vi "Configure Load Trigger Template.vi"(8 "error in (no error)":errorcluster, 9 "Arguments ()":string, 10 "Templates (0: ConfigList)":i32(ring) items=["ConfigList", "DurationLoop", "Empty", "GradeBinning", "Keithley2001", "LogicTrigger", "LoopUntilEvent", "SimpleLoop", "SortBinning"], 11 "VISA resource name":refnum<visa-resource-name>) -> (0 "error out":errorcluster, 3 "VISA resource name out":refnum<visa-resource-name>)   [LabVIEW 2020, in "Keithley DMM6500 DAQ6500 Series.lvlib"]
doc: "Load the trigger template with the arguments."
uses:
  <instrlib>/Keithley DMM6500 DAQ6500 Series/Keithley DMM6500 DAQ6500 Series.lvlib
panel:
  # "This VI is obsolete and these functions are \nincorporated in \"Configure Load Trigger Template.vi\""
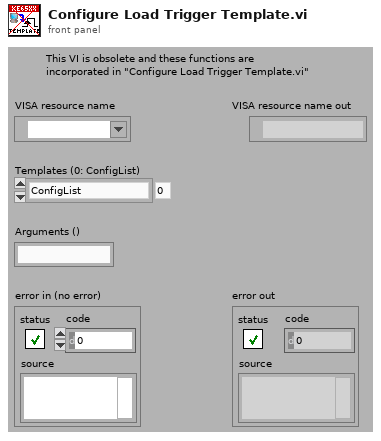
[diagram p1: front panel]
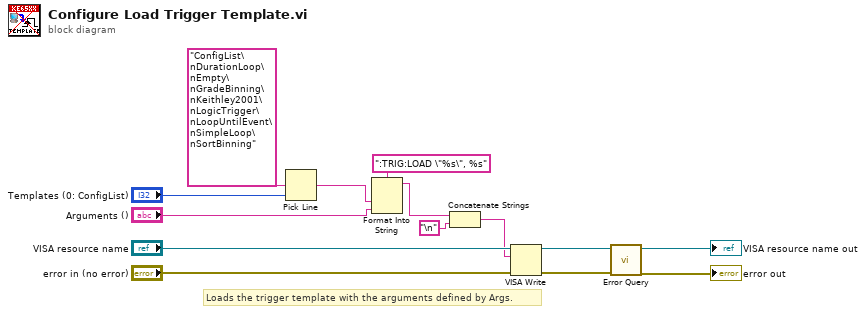
[diagram p0: block diagram]
diagram:
  # "Loads the trigger template with the arguments defined by Args."
  n1 = Pick Line(multi-line string="ConfigList\nDurationLoop\nEmpty\nGradeBinning\nKeithley2001\nLogicTrigger\nLoopUntilEvent\nSimpleLoop\nSortBinning", line index="Templates (0: ConfigList)") -> (output string=w7:string)  [unwired: 1 in]
  n2 = Format Into String(format string=":TRIG:LOAD \"%s\", %s", w7, "Arguments ()") -> (resulting string=w3:string)  [unwired: 2 in, 1 out]
  n3 = Concatenate Strings(w3, "\n") -> (w4:string)
  n4 = VISA Write(VISA resource name="VISA resource name", write buffer=w4, error in (no error)="error in (no error)") -> (VISA resource name out=w11:refnum<visa-resource-name>, error out=w10:errorcluster)  [unwired: 1 out]
  n5 = call <instrlib>:"Error Query.vi"("error in (no error)"=w10, "VISA resource name"=w11) -> ("error out"=→"error out":errorcluster, "VISA resource name out"=→"VISA resource name out":refnum<visa-resource-name>)  [unwired: 6 in, 2 out]
